vi "Write comment to file.vi"(6 "error in (no error)":errorcluster, 9 "refnum":refnum<file>) -> (0 "error out":errorcluster, 3 "dup refnum":refnum<file>)   [LabVIEW 2019]
panel:
  in  "Cancel Button":bool
  in  "OK Button":bool
  in  "Comment text to write in file":string
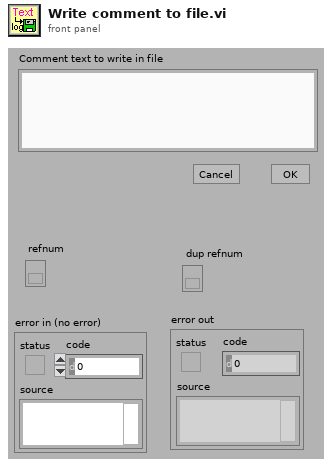
[diagram p1: front panel]
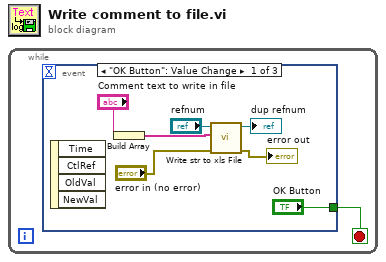
[diagram p0: block diagram]
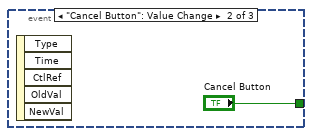
[diagram p2: hidden frame]
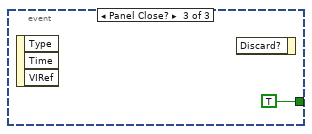
[diagram p3: hidden frame]
diagram:
  n1 = while {
    stop <- w1 stop-if-true
    n2 = event shown="[0] \"OK Button\": Value Change" {
      selector: _ -> [_ _ _]
      dyn-events: _ -> [_ _ _]
      timeout: _ -> [_ _ _]
      tunnel: ["OK Button" "Cancel Button" TRUE] -> w1
      event "OK Button": Value Change {
        n3 = event-data() -> ()  [unwired: 1 in, 4 out]
        n4 = Build Array("Comment text to write in file") -> (w5:string[])
        n5 = call "Write str to xls File.vi"("error in (no error)"="error in (no error)", "1D data"=w5, "refnum"="refnum") -> ("error out"=→"error out":errorcluster, "dup refnum"=→"dup refnum":refnum<file>)  [unwired: 7 in]
      }
      event "Cancel Button": Value Change {
        n6 = event-data() -> ()  [unwired: 1 in, 5 out]
      }
      event Panel Close? {
        n7 = event-data() -> ()  [unwired: 1 in, 3 out]
        n8 = event-data() -> ()  [unwired: 2 in, 1 out]
      }
    }
  }
